vi "Main.vi"   [LabVIEW 2020]
uses:
  Product/Color.ctl
  Product/Size.ctl
  BetterFilter/BetterFilter.lvclass
  BlahSpec/BlahSpec.lvclass
  C:/Repo/LabVIEW-SOLID-Examples/Examples/OCP/IFilterSpecification/IFilterSpecification.lvclass
  ColorSpecification/ColorSpecification.lvclass
  ColorSpecification/ColorSpecification.lvclass/ColorSpecification.ctl
  Product/Product.lvclass/Product.ctl
  ColorSpecification/Write Color.vi
  SizeSpecification/SizeSpecification.lvclass
  AndSpecification/AndSpecification.lvclass
  Product/Product.lvclass
  ProductFilter/ProductFilter.lvclass
types:
  T1 = typedef "Product.lvclass/Color.ctl" = enum16{"Blue", "Green", "Red"}
  T2 = typedef "Product.lvclass/Size.ctl" = enum16{"Yuge", "Big", "Medium", "Small"}
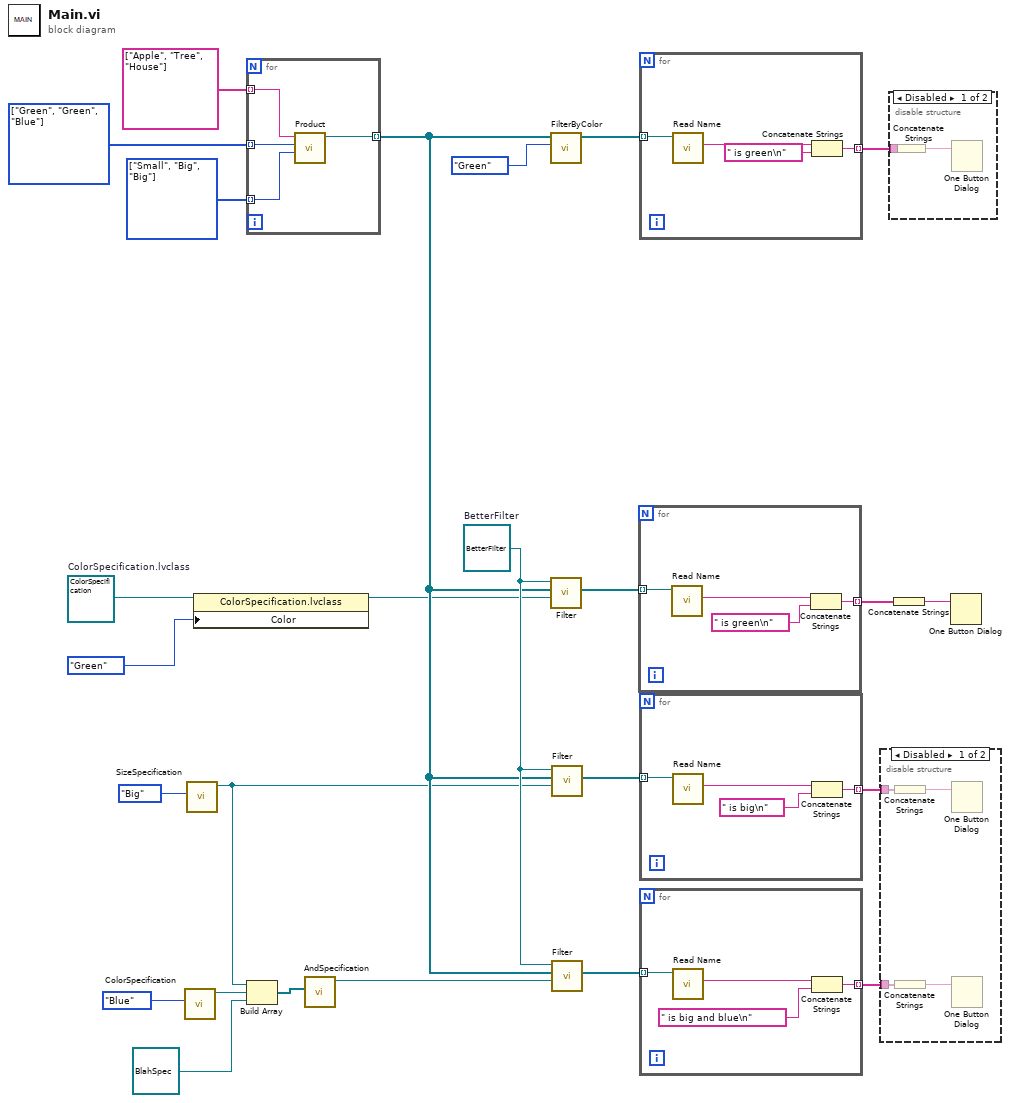
[diagram p0: block diagram]
diagram:
  w1 = refnum<class "ColorSpecification.lvclass"> refnum  # ColorSpecification.lvclass
  w11 = refnum<class "BetterFilter.lvclass"> refnum  # BetterFilter
  w23 = T2[] [enum."Small", enum."Big", enum."Big"] items=["Yuge", "Big", "Medium", "Small"] ("Array")
  w24 = T1[] [enum."Green", enum."Green", enum."Blue"] items=["Blue", "Green", "Red"] ("Array")
  n1 = call "ColorSpecification.vi"("Color"=Color."Blue") -> ("ColorSpecification"=w5:refnum<class "ColorSpecification.lvclass">)  [unwired: 10 in]
  n2 = call "SizeSpecification.vi"("Size"=Size."Big") -> ("SizeSpecification"=w9:refnum<class "SizeSpecification.lvclass">)  [unwired: 10 in]
  n3 = property class="ColorSpecification.lvclass"(reference=w1, "Color"=Color."Green") -> (reference out=w3:refnum<class "ColorSpecification.lvclass">)  [unwired: 1 in, 1 out]
  n4 = for {
    tunnel: string[] ["Apple", "Tree", "House"] ("Name") -> [w29] mode=indexing
    tunnel: w24 -> [w28] mode=indexing
    tunnel: w23 -> [w27] mode=indexing
    tunnel: [w26] -> w10 mode=indexing
    n5 = call "Product.vi"("Size"=w27, "Color"=w28, "Name"=w29) -> ("Product"=w26:refnum<class "Product.lvclass">)  [unwired: 8 in]
  }
  n6 = Build Array(w9, w5, refnum<class "BlahSpec.lvclass"> refnum ("BlahSpec.lvclass")) -> (w8:refnum<class "IFilterSpecification.lvclass">[])
  n7 = call "AndSpecification.vi"("Specifications"=w8) -> ("AndSpecification"=w7:refnum<class "AndSpecification.lvclass">)  [unwired: 10 in]
  n8 = call "FilterByColor.vi"("Color"=Color."Green", "Products In"=w10) -> ("Filtered Products"=w22:refnum<class "Product.lvclass">[])  [unwired: 9 in]
  n9 = call-dynamic "Filter.vi"("FilterSpecification"=w3, "Products In"=w10, "BetterFilter"=w11) -> ("Filtered Products"=w17:refnum<class "Product.lvclass">[])  [unwired: 8 in]
  n10 = call-dynamic "Filter.vi"("FilterSpecification"=w9, "Products In"=w10, "BetterFilter"=w11) -> ("Filtered Products"=w16:refnum<class "Product.lvclass">[])  [unwired: 8 in]
  n11 = call-dynamic "Filter.vi"("FilterSpecification"=w7, "Products In"=w10, "BetterFilter"=w11) -> ("Filtered Products"=w13:refnum<class "Product.lvclass">[])  [unwired: 8 in]
  n12 = for {
    tunnel: w17 -> [w33] mode=indexing
    tunnel: [w30] -> w18 mode=indexing
    n13 = call "Read Name.vi"("Product In"=w33) -> ("Name"=w32:string)  [unwired: 9 in, 1 out]
    n14 = Concatenate Strings(w32, " is green\n" ("string")) -> (w30:string)
  }
  n15 = for {
    tunnel: w22 -> [w37] mode=indexing
    tunnel: [w34] -> w20 mode=indexing
    n16 = call "Read Name.vi"("Product In"=w37) -> ("Name"=w36:string)  [unwired: 9 in, 1 out]
    n17 = Concatenate Strings(w36, " is green\n" ("string")) -> (w34:string)
  }
  n18 = for {
    tunnel: w16 -> [w41] mode=indexing
    tunnel: [w38] -> w15 mode=indexing
    n19 = call "Read Name.vi"("Product In"=w41) -> ("Name"=w40:string)  [unwired: 9 in, 1 out]
    n20 = Concatenate Strings(w40, " is big\n" ("string")) -> (w38:string)
  }
  n21 = for {
    tunnel: w13 -> [w45] mode=indexing
    tunnel: [w42] -> w14 mode=indexing
    n22 = call "Read Name.vi"("Product In"=w45) -> ("Name"=w44:string)  [unwired: 9 in, 1 out]
    n23 = Concatenate Strings(w44, " is big and blue\n" ("string")) -> (w42:string)
  }
  n24 = disable-structure shown="Disabled" {
    disable-tunnel: w15 -> [w49 _]
    disable-tunnel: w14 -> [w46 _]
    frame Disabled {
      n25 = Concatenate Strings(w49) -> (w48:string)
      n26 = Concatenate Strings(w46) -> (w47:string)
      n27 = One Button Dialog(message=w48) -> ()  [unwired: 1 in, 1 out]
      n28 = One Button Dialog(message=w47) -> ()  [unwired: 1 in, 1 out]
    }
    frame Enabled {
    }
  }
  n29 = disable-structure shown="Disabled" {
    disable-tunnel: w20 -> [w51 _]
    frame Disabled {
      n30 = Concatenate Strings(w51) -> (w50:string)
      n31 = One Button Dialog(message=w50) -> ()  [unwired: 1 in, 1 out]
    }
    frame Enabled {
    }
  }
  n32 = Concatenate Strings(w18) -> (w19:string)
  n33 = One Button Dialog(message=w19) -> ()  [unwired: 1 in, 1 out]
